vi "ISEG_HVBoard.contents.vi"   [LabVIEW 2014, in "ISEG_HVBoard.lvlib"]
doc: "loads all VIs of a class into memory - required for building applications"
uses:
  ISEG_HVBoard.lvlib
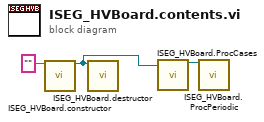
[diagram p0: block diagram]
diagram:
  n1 = call "ISEG_HVBoard.constructor.vi"("name"="") -> ("i ref out"=w2:refnum<vi>)  [unwired: 16 in, 2 out]
  n2 = call "ISEG_HVBoard.destructor.vi"("i ref in"=w2) -> ()  [unwired: 18 in, 1 out]
  n3 = call "ISEG_HVBoard.ProcCases.vi"("i ref in"=w2) -> ("i ref out"=w1:refnum<vi>)  [unwired: 16 in, 2 out]
  n4 = call "ISEG_HVBoard.ProcPeriodic.vi"("i ref in"=w1) -> ()  [unwired: 16 in, 3 out]
